vi "Set OP and Post OP Measurements.vi"(8 "error in (no error)":errorcluster, 11 "Servo to Compression in":refnum<class "Servo to Compression.lvclass">) -> (0 "error out":errorcluster, 3 "Servo to Compression out":refnum<class "Servo to Compression.lvclass">)   [LabVIEW 2018, in "Servo to Compression.lvlib" / "Servo to Compression.lvclass"]
uses:
  Servo to Compression.lvclass
  Plugins/Measurements/Servo MSMT.lvlibp/Servo MSMT.lvclass
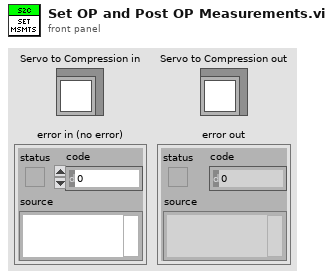
[diagram p1: front panel]
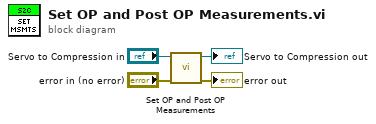
[diagram p0: block diagram]
diagram:
  n1 = call-parent "Set OP and Post OP Measurements.vi"("error in (no error)"="error in (no error)", "Servo MSMT in"="Servo to Compression in") -> ("error out"=→"error out":errorcluster, "Servo MSMT out"=→"Servo to Compression out":refnum<class "Servo to Compression.lvclass">)  [unwired: 8 in]
